vi "LIA Example FPGA.vi"() -> ()   [LabVIEW 2017]
uses:
  <instrlib>/_niInstr/Streaming/v1/Common/Stream State.ctl
  <instrlib>/_niInstr/Data Trigger/v1/Shared/Public/Edge Configuration FXP(+-,18,1).ctl
  <instrlib>/_niInstr/Data Trigger/v1/Shared/Public/Edge Configuration Trigger Slope.ctl
  <vilib>/Platform/TimedLoop/XDataNode/timing_clust.ctl
  <vilib>/Platform/TimedLoop/XDataNode/nitl_modes.ctl
  <vilib>/Platform/TimedLoop/XDataNode/wakeup.ctl
  <instrlib>/_niInstr/DSP/v1/Shared/Public/IQ Data.ctl
  <vilib>/rvi/Emulation/niFpgaSctlEmulationGetInTimedLoop.vi
  <vilib>/rvi/Emulation/niFpgaEmulationReportErrorSimple.vi
  <vilib>/rvi/Emulation/niFpgaGetClockAttributes.vi
  <vilib>/rvi/Emulation/niFpgaCriticalErrorInLSC.vi
  <instrlib>/_niInstr/DSP/v1/FPGA/Public/Sub VIs/Frequency Shift/Frequency Shift - 1 spc.vi
  <instrlib>/_niInstr/DSP/v1/FPGA/Public/Sub VIs/Fractional Decimator/Fractional Decimator - 1 spc - 2x oc.vi
  <userlib>/_NI Noise Generation IP/FPGA/Public/Low Level/AWGN FXP23x2.vi
  <instrlib>/_niInstr/DSP/v1/FPGA/Public/Sub VIs/Frequency Shift/Frequency Shift - 2 spc.vi
  <vilib>/rvi/eio/common/nirviEmuTemplateMethod_errors.vi
  <vilib>/Platform/TimedLoop/XDataNode/XDataNode.xnode
  <instrlib>/_niInstr/DSP/v1/Xnodes/Public/Frequency Shift/niInstr DSP v1 Frequency Shift FPGA.xnode
  <vilib>/rvi/FXPMathLib/FxpMul/XNode/nifxpmath_Multiplier.xnode
  <vilib>/rvi/FXPMathLib/FxpAdd/XNode/nifxpmath_Add.xnode
  <vilib>/eio/EIONode/EIONode.xnode
  <vilib>/Platform/TimedLoop/XDataNode/XDNodeRunTimeDep.lvlib
  <instrlib>/_niInstr/Basic Elements/v1/FPGA/niInstr Basic Elements v1 FPGA.lvlib
  <instrlib>/_niInstr/DSP/v1/Shared/niInstr DSP v1 Shared.lvlib
  <instrlib>/_niInstr/DSP/v1/FPGA/niInstr DSP v1 FPGA.lvlib
  Program Files (x86)/National Instruments/LabVIEW 2017/examples/Lock-In Amplifier/_NI PLL IP/FPGA/NI PLL IP FPGA.lvlib
  lib/fpga/Lock-In Amplifier Example FPGA.lvlib
  <instrlib>/_niInstr/Streaming/v1/Common/niInstr Streaming v1 Common.lvlib
  <userlib>/_NI Noise Generation IP/FPGA/NI Noise Generation IP FPGA v2.lvlib
  <vilib>/rvi/FXPMathLib/sim/FxpSim.dll
  <instrlib>/_niInstr/Data Trigger/v1/Shared/niInstr Data Trigger v1 Shared.lvlib
panel:
  in  "lock-in.fir fs":fxp<+,48,1>
  in  "lock-in.decimator 0":enum16{"CIC", "FIR"}(ring)
  in  "dpll.reset 1":bool
  in  "dpll.enable 1":bool
  in  "dpll.q 1":fxp<+,48,0>
  in  "dpll.m 1":i8
  in  "dpll.config 1":T1
  out "dpll.vco output 1":fxp<+/-,48,0>
  in  "dpll.channel 1":i32
  in  "dpll.channel 0":i32
  out "dpll.vco output 0":fxp<+/-,48,0>
  in  "dpll.config 0":T1
  in  "dpll.m 0":i8
  in  "dpll.q 0":fxp<+,48,0>
  in  "dpll.enable 0":bool
  in  "dpll.reset 0":bool
  in  "lock-in.enable 3":bool
  in  "lock-in.enable 2":bool
  in  "lock-in.enable 1":bool
  in  "lock-in.carrier 3":fxp<+/-,48,0>
  in  "lock-in.carrier 2":fxp<+/-,48,0>
  in  "lock-in.enable 0":bool
  in  "lock-in.channel select 3":i32
  in  "lock-in.carrier select 3":i32
  in  "lock-in.cic config valid 3":bool
  in  "lock-in.cic config 3":cluster{"factor":fxp<+,16,16>, "shift":i16}
  in  "lock-in.reset 3":bool
  out "stream.state 3":T3 caption="stream.state 0"
  out "stream.samples transferred 3":u64 caption="stream.samples transferred 0"
  out "stream.metadata 3":u64 caption="stream.metadata 0"
  in  "stream.num samples 3":u64 caption="stream.num samples 0"
  in  "stream.request state 3":T3 caption="stream.request state 0"
  in  "lock-in.channel select 2":i32
  in  "lock-in.carrier select 2":i32
  in  "lock-in.cic config valid 2":bool
  in  "lock-in.cic config 2":cluster{"factor":fxp<+,16,16>, "shift":i16}
  in  "lock-in.reset 2":bool
  out "stream.state 2":T3 caption="stream.state 0"
  out "stream.samples transferred 2":u64 caption="stream.samples transferred 0"
  out "stream.metadata 2":u64 caption="stream.metadata 0"
  in  "stream.num samples 2":u64 caption="stream.num samples 0"
  in  "stream.request state 2":T3 caption="stream.request state 0"
  out "pll.vco output 0":fxp<+/-,48,0>
  out "pll.vco output 1":fxp<+/-,48,0>
  out "stream.metadata 4":u64 caption="stream.metadata 0"
  out "stream.samples transferred 4":u64 caption="stream.samples transferred 0"
  out "stream.state 4":T3 caption="stream.state 0"
  in  "stream.request state 4":T3 caption="stream.request state 0"
  in  "stream.num samples 4":u64 caption="stream.num samples 0"
  in  "preview.channel select":i32
  in  "ao.reset 3":bool
  in  "ao.carrier 2":fxp<+/-,48,0>=0.010000000000001563
  in  "ao.level 2":fxp<+/-,18,1>
  in  "ao.reset 2":bool
  in  "ao.carrier 1":fxp<+/-,48,0>=0.010000000000001563
  in  "ao.level 1":fxp<+/-,18,1>
  in  "ao.reset 1":bool
  in  "ao.reset 0":bool
  in  "ao.carrier 0":fxp<+/-,48,0>=0.010000000000001563
  in  "ao.level 0":fxp<+/-,18,1>
  in  "lock-in.channel select 1":i32
  in  "lock-in.channel select 0":i32
  in  "stream.request state 1":T3 caption="stream.request state 0"
  in  "stream.num samples 1":u64 caption="stream.num samples 0"
  out "stream.metadata 1":u64 caption="stream.metadata 0"
  out "stream.samples transferred 1":u64 caption="stream.samples transferred 0"
  out "stream.state 1":T3 caption="stream.state 0"
  in  "lock-in.reset 1":bool
  in  "lock-in.cic config 1":cluster{"factor":fxp<+,16,16>, "shift":i16}
  in  "lock-in.cic config valid 1":bool
  in  "lock-in.carrier select 1":i32
  in  "lock-in.carrier select 0":i32
  in  "lock-in.cic config valid 0":bool
  in  "lock-in.cic config 0":cluster{"factor":fxp<+,16,16>, "shift":i16}
  in  "lock-in.reset 0":bool
  in  "lock-in.carrier 1":fxp<+/-,48,0>
  in  "lock-in.carrier 0":fxp<+/-,48,0>
  in  "ao.level 3":fxp<+/-,18,1>
  in  "pll.channel 1":i32
  in  "pll.reset 1":bool
  in  "pll.enable 1":bool
  in  "pll.config 1":T4={"quiescent frequency"=0.10000000000000142, "compensation"=0.0, "psd gain"=-18, "loop filter"={"order"=4, "cutoff"=6}}
  in  "pll.channel 0":i32
  in  "ao.noise gain 3":fxp<+,18,1>=0.01000213623046875
  in  "ao.carrier 3":fxp<+/-,48,0>=0.010000000000001563
  in  "ao.noise seeds 3":fxp<+,23,23>[](array[numeric])=[1.0, 12323.0]
  in  "pll.reset 0":bool
  in  "pll.enable 0":bool
  in  "stream.request state 0":T3
  in  "stream.num samples 0":u64
  out "stream.metadata 0":u64
  out "stream.samples transferred 0":u64
  out "stream.state 0":T3
  in  "pll.config 0":T4={"quiescent frequency"=0.10000000000000142, "compensation"=0.0, "psd gain"=-18, "loop filter"={"order"=4, "cutoff"=6}}
  out "IO Module\\InitDone":bool
  out "IO Module\\User Error":u32
  in  "IO Module\\User Command":u32
  in  "IO Module\\User Command Valid":bool
  out "IO Module\\User Command Ready":bool
  in  "IO Module\\User Command Arg 0":u32
  in  "IO Module\\User Command Arg 1":u32
  out "IO Module\\User Command Error":u16
  out "IO Module\\User Command Return":u32
  out "IO Module\\User Command Return Valid":bool
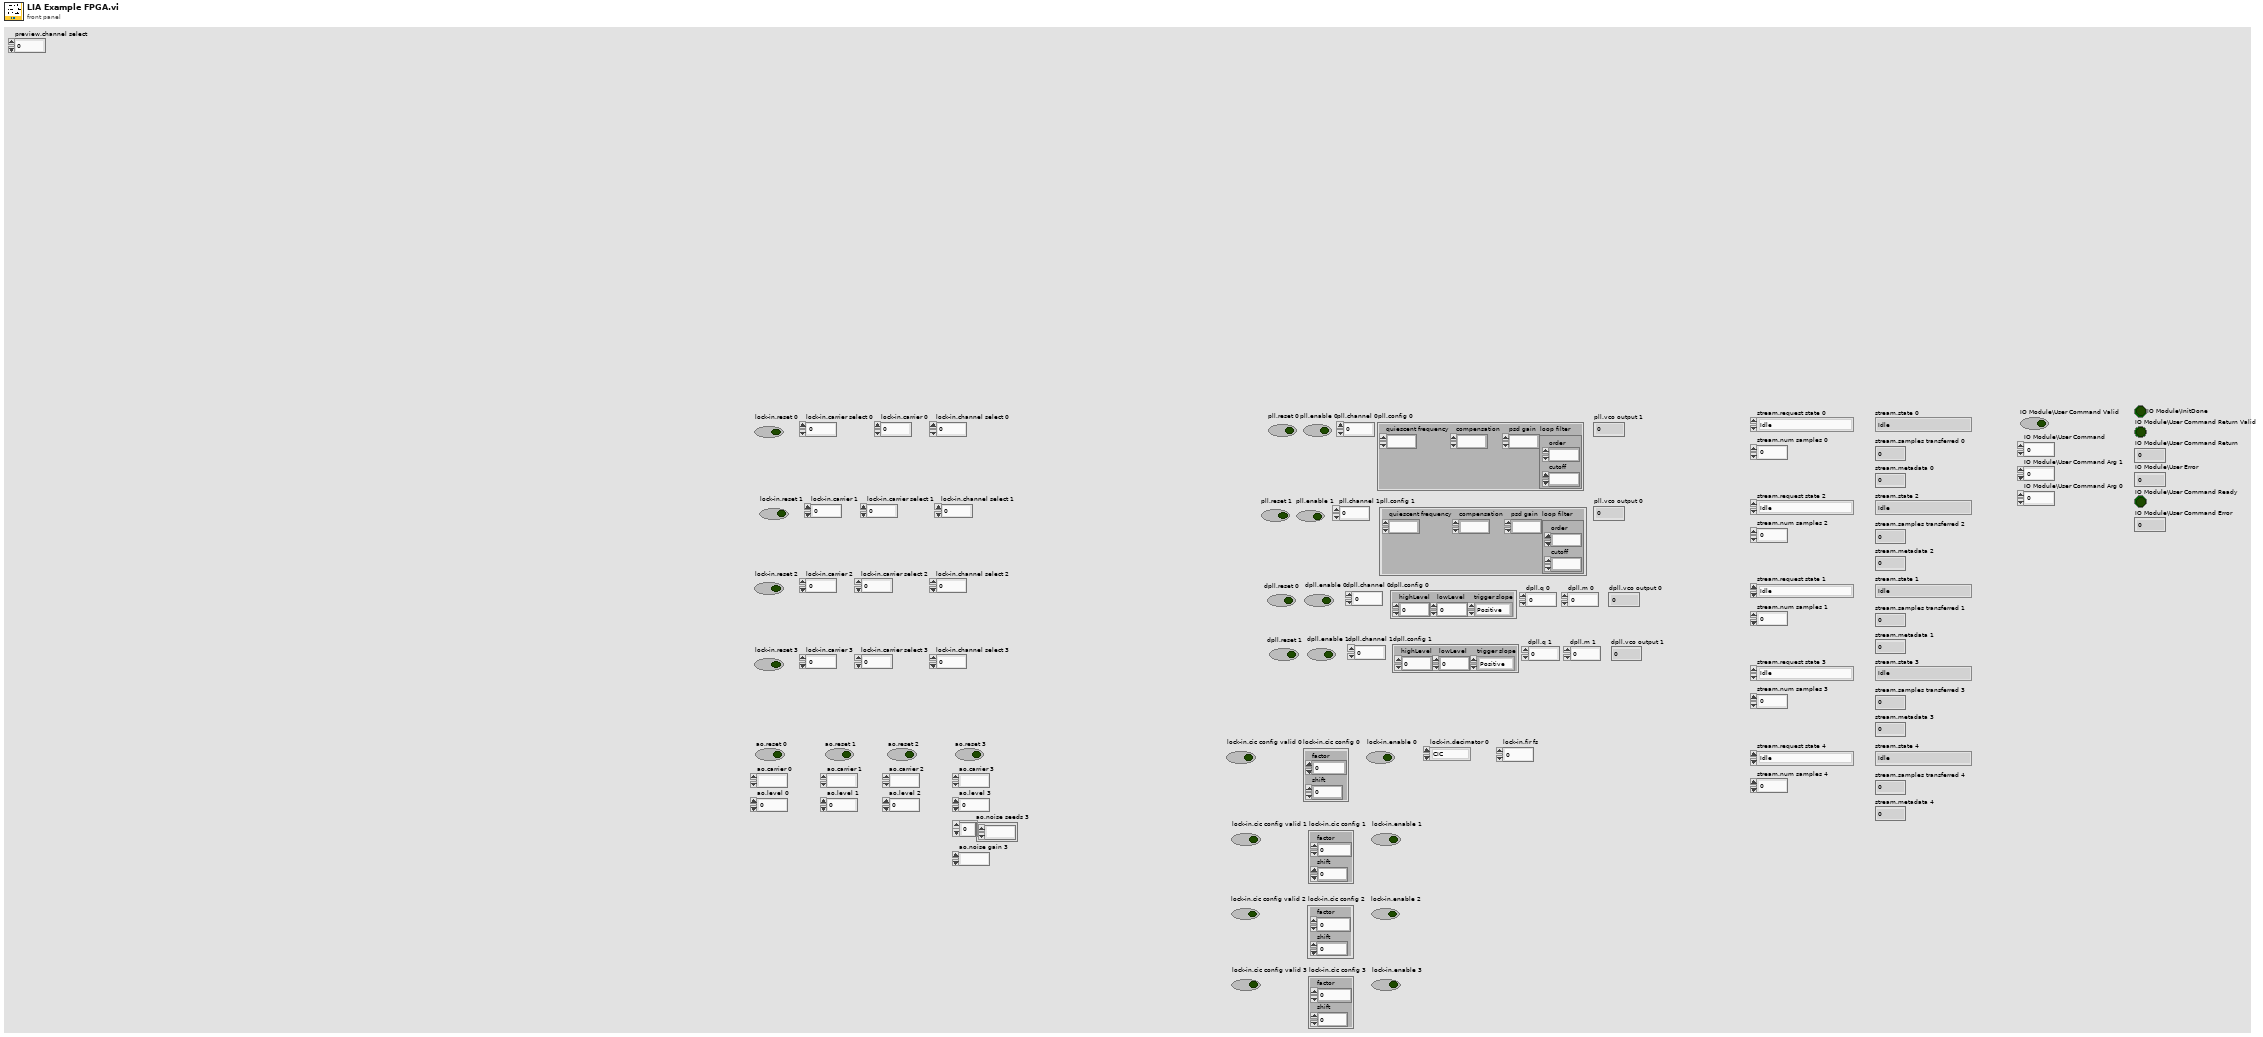
[diagram p1: front panel]
types:
  T1 = typedef "niInstr Data Trigger v1 Shared.lvlib/Edge Configuration FXP(+-,18,1).ctl" = cluster{"highLevel":fxp<+/-,18,1>, "lowLevel":fxp<+/-,18,1>, "trigger slope":T2}
  T2 = typedef "niInstr Data Trigger v1 Shared.lvlib/Edge Configuration Trigger Slope.ctl" = enum8{"Positive", "Negative"}
  T3 = typedef "niInstr Streaming v1 Common.lvlib/Stream State.ctl" = enum8{"Idle", "Finite Transfer", "Continuous", "Done", "Error", "Not Ready", "Cancel"}
  T4 = cluster{"quiescent frequency":fxp<+/-,48,0>, "compensation":fxp<+/-,18,3>, "psd gain":i16, "loop filter":cluster{"order":i32, "cutoff":i8}}
  T5 = typedef "XDNodeRunTimeDep.lvlib/timing_clust.ctl" = cluster{"Expected End [f-1]":u64, "Actual End [f-1]":u64, "Finished Late? [f-1]":bool, "Expected End [i-1]":u64, "Actual End [i-1]":u64, "Finished Late? [i-1]":bool, "Expected Start [i]":u64, "Actual Start [i]":u64, "Expected Start [f]":u64, "Actual Start [f]":u64, "Source Name":string, "Structure Name":string, "Period":i64, "Deadline":i64, "Offset":i64, "Start":i64, "Priority":i32, "Timeout":i32, "Mode":T6, "Wakeup Reason":T7, "Error":errorcluster, "Source Type":string, "Secondary Source Type":string, "Global End Time":u64, "Global Start Time":u64, "Frame Duration":u64, "Iteration Duration":u64, "Assigned CPU":i32, "I/O Scan Engine Mode":u32}
  T6 = typedef "XDNodeRunTimeDep.lvlib/nitl_modes.ctl" = enum32{"No Change", "Process missed periods, maintain original phase", "Discard missed periods, maintain original phase", "Process missed periods, ignore original phase", "Discard missed periods, ignore original phase"}
  T7 = typedef "XDNodeRunTimeDep.lvlib/wakeup.ctl" = enum32{"Normal", "Aborted", "Asynchronous wakeup", "Timing source error", "Timed loop error", "Timeout"}
  T8 = cluster{"stream.num samples 0":u64, "stream.request state 0":T3, "stream.index 0":i16}
  T9 = typedef "niInstr DSP v1 Shared.lvlib/IQ Data.ctl" = cluster{"I":fxp<+/-,18,1>, "Q":fxp<+/-,18,1>, "overflow":bool}
  T10 = cluster{"stream.metadata 0":u64, "stream.samples transferred 0":u64, "stream.state 0":T3}
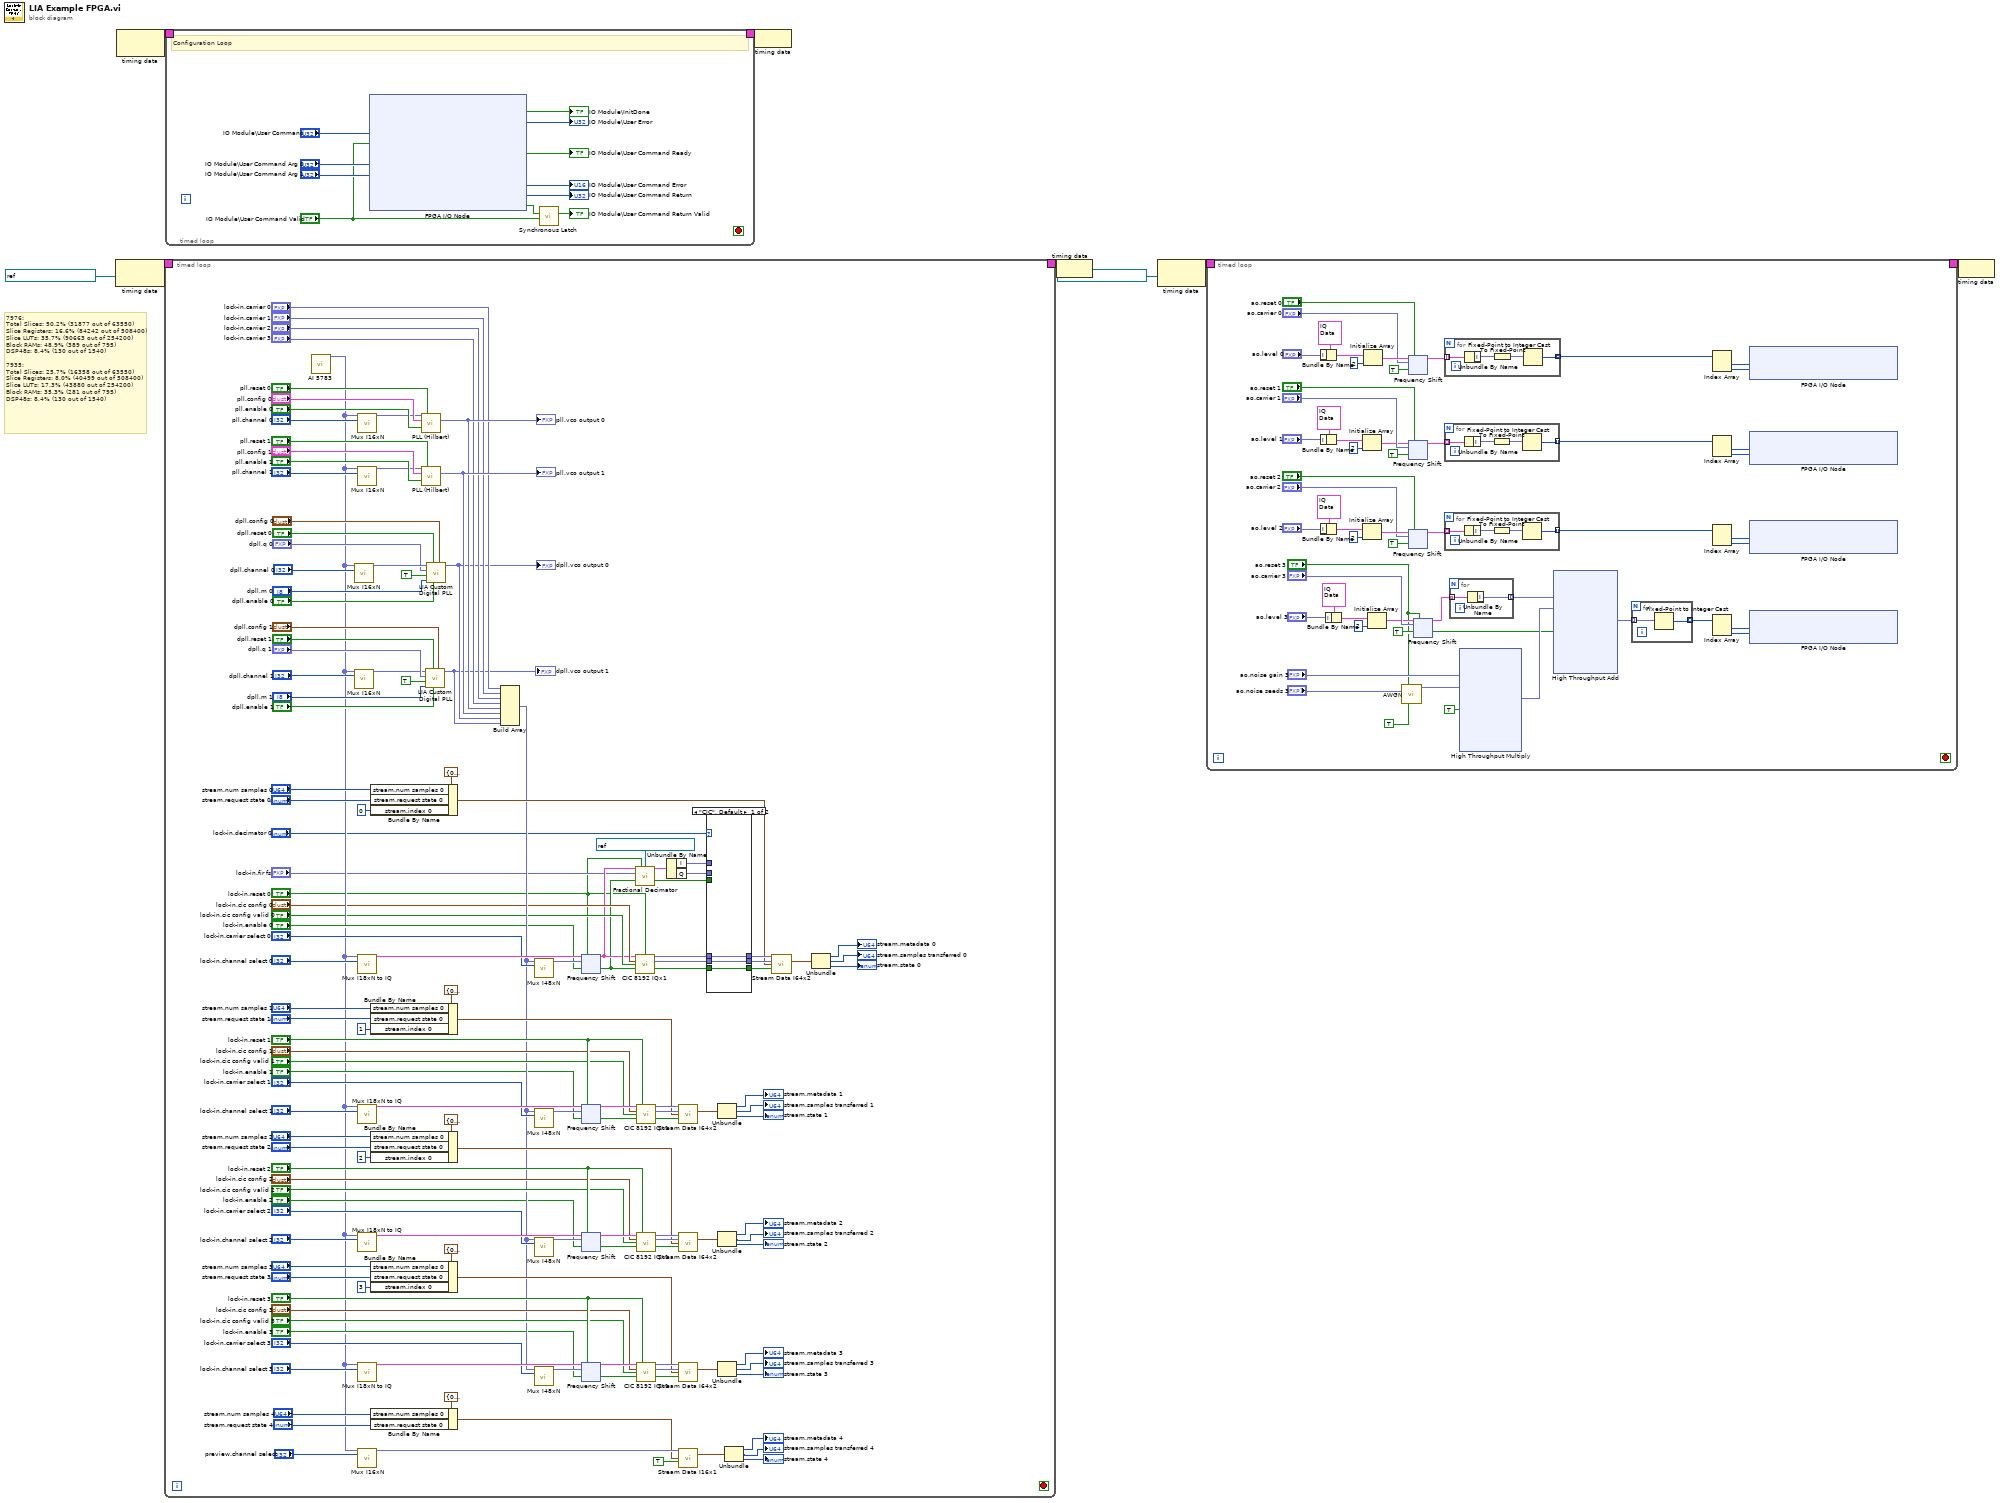
[diagram p0: block diagram]
diagram:
  # "7976:\nTotal Slices: 50.2% (31877 out of 63550)\nSlice Registers: 16.6% (84242 out of 508400)\nSlice LUTs: 35.7% (90663 out of 254200)\nBlock RAMs: 48.9% (389 out of 795)\nDSP48s: 8.4% (130 out of 1540)\n\n7935:\nTotal Slices: 25.7% (16358 out of 63550)\nSlice Registers: 8.0% (40499 out of 508400)\nSlice LUTs: 17.3% (43880 out of 254200)\nBlock RAMs: 35.3% (281 out of 795)\nDSP48s: 8.4% (130 out of 1540)"
  n1 = node-c288(refnum<k21> "IO Module\\Data Clock" ("Source Name")) -> (w8:T5)
  n2 = node-c288() -> (w2:T5)  [unwired: 1 in]
  n3 = timed-loop {
    timing: w8 -> [_]
    timing-out: [_] -> w7
    stop <- _ stop-if-true
    n4 = call "AI 5783.vi"() -> ("i18x1"=w25:fxp<+/-,18,1>[])  [unwired: 14 in, 1 out]
    n5 = call "Mux I16xN.vi"("i16xn in"=w25, "index"="dpll.channel 1") -> ("i16 out"=w28:fxp<+/-,18,1>)  [unwired: 12 in, 1 out]
    n6 = call "Mux I16xN.vi"("i16xn in"=w25, "index"="dpll.channel 0") -> ("i16 out"=w40:fxp<+/-,18,1>)  [unwired: 12 in, 1 out]
    n7 = call "Mux I16xN.vi"("i16xn in"=w25, "index"="pll.channel 0") -> ("i16 out"=w150:fxp<+/-,18,1>)  [unwired: 12 in, 1 out]
    n8 = call "Mux I16xN.vi"("i16xn in"=w25, "index"="pll.channel 1") -> ("i16 out"=w144:fxp<+/-,18,1>)  [unwired: 12 in, 1 out]
    n9 = call "Mux I18xN to IQ.vi"("i16xn in"=w25, "index"="lock-in.channel select 0") -> ("output"=w143:T9)  [unwired: 12 in, 1 out]
    n10 = call "Mux I18xN to IQ.vi"("i16xn in"=w25, "index"="lock-in.channel select 1") -> ("output"=w127:T9)  [unwired: 12 in, 1 out]
    n11 = call "Mux I18xN to IQ.vi"("i16xn in"=w25, "index"="lock-in.channel select 2") -> ("output"=w93:T9)  [unwired: 12 in, 1 out]
    n12 = call "Mux I18xN to IQ.vi"("i16xn in"=w25, "index"="lock-in.channel select 3") -> ("output"=w72:T9)  [unwired: 12 in, 1 out]
    n13 = call "Mux I16xN.vi"("i16xn in"=w25, "index"="preview.channel select") -> ("i16 out"=w101:fxp<+/-,18,1>)  [unwired: 12 in, 1 out]
    n14 = Bundle By Name(cluster=T8 {"stream.num samples 0"=0, "stream.request state 0"=enum."Idle", "stream.index 0"=0} ("config"), "stream.num samples 0"="stream.num samples 0", "stream.request state 0"="stream.request state 0", "stream.index 0"=i16 0) -> (w130:T8)
    n15 = Bundle By Name(cluster=T8 {"stream.num samples 0"=0, "stream.request state 0"=enum."Idle", "stream.index 0"=0} ("config"), "stream.num samples 0"="stream.num samples 1", "stream.request state 0"="stream.request state 1", "stream.index 0"=i16 1) -> (w109:T8)
    n16 = Bundle By Name(cluster=T8 {"stream.num samples 0"=0, "stream.request state 0"=enum."Idle", "stream.index 0"=0} ("config"), "stream.num samples 0"="stream.num samples 2", "stream.request state 0"="stream.request state 2", "stream.index 0"=i16 2) -> (w75:T8)
    n17 = Bundle By Name(cluster=T8 {"stream.num samples 0"=0, "stream.request state 0"=enum."Idle", "stream.index 0"=0} ("config"), "stream.num samples 0"="stream.num samples 3", "stream.request state 0"="stream.request state 3", "stream.index 0"=i16 3) -> (w54:T8)
    n18 = Bundle By Name(cluster=T8 {"stream.num samples 0"=0, "stream.request state 0"=enum."Idle", "stream.index 0"=0} ("config"), "stream.num samples 0"="stream.num samples 4", "stream.request state 0"="stream.request state 4") -> (w97:T8)
    n19 = call "PLL (Hilbert).vi"("input"=w150, "reset"="pll.reset 0", "config"="pll.config 0", "enable"="pll.enable 0") -> ("output"=w94:fxp<+/-,48,0>)  [unwired: 11 in]
    "pll.vco output 0" <- w94
    n20 = call "PLL (Hilbert).vi"("input"=w144, "reset"="pll.reset 1", "config"="pll.config 1", "enable"="pll.enable 1") -> ("output"=w95:fxp<+/-,48,0>)  [unwired: 11 in]
    "pll.vco output 1" <- w95
    n21 = call "LIA Custom Digital PLL.vi"("configuration"="dpll.config 1", "arm"="dpll.enable 1", "reset"="dpll.reset 1", "m"="dpll.m 1", "input valid"=TRUE, "q"="dpll.q 1", "I"=w28) -> ("frequency shift"=w24:fxp<+/-,48,0>)  [unwired: 1 in, 3 out]
    "dpll.vco output 1" <- w24
    n22 = call "LIA Custom Digital PLL.vi"("configuration"="dpll.config 0", "arm"="dpll.enable 0", "reset"="dpll.reset 0", "m"="dpll.m 0", "input valid"=TRUE, "q"="dpll.q 0", "I"=w40) -> ("frequency shift"=w35:fxp<+/-,48,0>)  [unwired: 1 in, 3 out]
    "dpll.vco output 0" <- w35
    n23 = Build Array("lock-in.carrier 0", "lock-in.carrier 1", "lock-in.carrier 2", "lock-in.carrier 3", w94, w95, w35, w24) -> (w51:fxp<+/-,48,0>[])
    n24 = call "Mux I48xN.vi"("i48xn in"=w51, "index"="lock-in.carrier select 0") -> ("i48 out"=w142:fxp<+/-,48,0>)  [unwired: 13 in]
    n25 = call "Mux I48xN.vi"("i48xn in"=w51, "index"="lock-in.carrier select 1") -> ("i48 out"=w126:fxp<+/-,48,0>)  [unwired: 13 in]
    n26 = call "Mux I48xN.vi"("i48xn in"=w51, "index"="lock-in.carrier select 2") -> ("i48 out"=w92:fxp<+/-,48,0>)  [unwired: 13 in]
    n27 = call "Mux I48xN.vi"("i48xn in"=w51, "index"="lock-in.carrier select 3") -> ("i48 out"=w71:fxp<+/-,48,0>)  [unwired: 13 in]
    n28 = xnode "Frequency Shift"("data in"=w143, "reset"="lock-in.reset 0", "frequency shift"=w142, "input valid"="lock-in.enable 0") -> ("data out"=w18:T9, "output valid"=w13:bool)  [unwired: 2 in, 1 out]
    n29 = xnode "Frequency Shift"("data in"=w127, "reset"="lock-in.reset 1", "frequency shift"=w126, "input valid"="lock-in.enable 1") -> ("data out"=w125:T9, "output valid"=w124:bool)  [unwired: 2 in, 1 out]
    n30 = xnode "Frequency Shift"("data in"=w93, "reset"="lock-in.reset 2", "frequency shift"=w92, "input valid"="lock-in.enable 2") -> ("data out"=w91:T9, "output valid"=w90:bool)  [unwired: 2 in, 1 out]
    n31 = xnode "Frequency Shift"("data in"=w72, "reset"="lock-in.reset 3", "frequency shift"=w71, "input valid"="lock-in.enable 3") -> ("data out"=w70:T9, "output valid"=w69:bool)  [unwired: 2 in, 1 out]
    n32 = call-poly <instrlib>:"Fractional Decimator.vi"("data in"=w18, "reset"="lock-in.reset 0", "clock x 2"=refnum<k21> "IO Module\\Data Clock 2x", "output sample rate"="lock-in.fir fs", "input valid"=w13) -> ("data out"=w21:T9, "output valid"=w10:bool)  [unwired: 8 in, 1 out]
    n33 = call "CIC 8192 IQx1.vi"("data"=w18, "reset"="lock-in.reset 0", "config"="lock-in.cic config 0", "config valid"="lock-in.cic config valid 0", "input valid"=w13) -> ("i out"=w17:fxp<+/-,64,1>, "q out"=w16:fxp<+/-,64,1>, "output valid"=w15:bool)  [unwired: 8 in]
    n34 = call "CIC 8192 IQx1.vi"("data"=w125, "reset"="lock-in.reset 1", "config"="lock-in.cic config 1", "config valid"="lock-in.cic config valid 1", "input valid"=w124) -> ("i out"=w120:fxp<+/-,64,1>, "q out"=w119:fxp<+/-,64,1>, "output valid"=w118:bool)  [unwired: 8 in]
    n35 = call "CIC 8192 IQx1.vi"("data"=w91, "reset"="lock-in.reset 2", "config"="lock-in.cic config 2", "config valid"="lock-in.cic config valid 2", "input valid"=w90) -> ("i out"=w86:fxp<+/-,64,1>, "q out"=w85:fxp<+/-,64,1>, "output valid"=w84:bool)  [unwired: 8 in]
    n36 = call "CIC 8192 IQx1.vi"("data"=w70, "reset"="lock-in.reset 3", "config"="lock-in.cic config 3", "config valid"="lock-in.cic config valid 3", "input valid"=w69) -> ("i out"=w65:fxp<+/-,64,1>, "q out"=w64:fxp<+/-,64,1>, "output valid"=w63:bool)  [unwired: 8 in]
    n37 = Unbundle By Name(w21) -> ("I"=w11:fxp<+/-,18,1>, "Q"=w9:fxp<+/-,18,1>)
    n38 = call "Stream Data I64x2.vi"("i in"=w120, "q in"=w119, "config"=w109, "input valid"=w118) -> ("status"=w117:T10)  [unwired: 11 in]
    n39 = call "Stream Data I64x2.vi"("i in"=w86, "q in"=w85, "config"=w75, "input valid"=w84) -> ("status"=w83:T10)  [unwired: 11 in]
    n40 = call "Stream Data I64x2.vi"("i in"=w65, "q in"=w64, "config"=w54, "input valid"=w63) -> ("status"=w62:T10)  [unwired: 11 in]
    n41 = call "Stream Data I16x1.vi"("i in"=w101, "config"=w97, "input valid"=TRUE) -> ("status"=w103:T10)  [unwired: 12 in]
    n42 = case shown="\"CIC\", Default" "lock-in.decimator 0" {
      tunnel: [w156 w159] -> w141
      tunnel: [w155 w158] -> w140
      tunnel: [w154 w157] -> w139
      tunnel: w17 -> [w156 _]
      tunnel: w16 -> [w155 _]
      tunnel: w15 -> [w154 _]
      tunnel: w11 -> [_ w159]
      tunnel: w10 -> [_ w157]
      tunnel: w9 -> [_ w158]
      frame "CIC", Default {
      }
      frame "FIR" {
      }
    }
    n43 = Unbundle(w117) -> ("stream.metadata 0"=→"stream.metadata 1":u64, "stream.samples transferred 0"=→"stream.samples transferred 1":u64, "stream.state 0"=→"stream.state 1":T3)
    n44 = Unbundle(w83) -> ("stream.metadata 0"=→"stream.metadata 2":u64, "stream.samples transferred 0"=→"stream.samples transferred 2":u64, "stream.state 0"=→"stream.state 2":T3)
    n45 = Unbundle(w62) -> ("stream.metadata 0"=→"stream.metadata 3":u64, "stream.samples transferred 0"=→"stream.samples transferred 3":u64, "stream.state 0"=→"stream.state 3":T3)
    n46 = Unbundle(w103) -> ("stream.metadata 0"=→"stream.metadata 4":u64, "stream.samples transferred 0"=→"stream.samples transferred 4":u64, "stream.state 0"=→"stream.state 4":T3)
    n47 = call "Stream Data I64x2.vi"("i in"=w141, "q in"=w140, "config"=w130, "input valid"=w139) -> ("status"=w138:T10)  [unwired: 11 in]
    n48 = Unbundle(w138) -> ("stream.metadata 0"=→"stream.metadata 0":u64, "stream.samples transferred 0"=→"stream.samples transferred 0":u64, "stream.state 0"=→"stream.state 0":T3)
  }
  n49 = timed-loop {
    timing: w2 -> [_]
    timing-out: [_] -> w1
    stop <- _ stop-if-true
    # "Configuration Loop"
    n50 = xnode "FPGA I/O Node"("IO Module\\User Command"="IO Module\\User Command", "IO Module\\User Command Valid"="IO Module\\User Command Valid", "IO Module\\User Command Arg 0"="IO Module\\User Command Arg 0", "IO Module\\User Command Arg 1"="IO Module\\User Command Arg 1") -> ("IO Module\\InitDone"=→"IO Module\\InitDone":bool, "IO Module\\Clip Error Code"=→"IO Module\\User Error":u32, "IO Module\\User Command Ready"=→"IO Module\\User Command Ready":bool, "IO Module\\User Command Error"=→"IO Module\\User Command Error":u16, "IO Module\\User Command Return"=→"IO Module\\User Command Return":u32, "IO Module\\User Command Return Valid"=w199:bool)  [unwired: 10 in, 10 out]
    n51 = call <instrlib>:"Synchronous Latch.vi"("clear"="IO Module\\User Command Valid", "set"=w199) -> ("out"=→"IO Module\\User Command Return Valid":bool)  [unwired: 9 in]
  }
  n52 = node-c288(w1) -> ()
  n53 = node-c288(w7) -> ()
  n54 = node-c288(refnum<k21> "IO Module\\Data Clock" ("Source Name")) -> (w5:T5)
  n55 = timed-loop {
    timing: w5 -> [_]
    timing-out: [_] -> w4
    stop <- _ stop-if-true
    n56 = Bundle By Name(cluster=T9 {"I"=0.0, "Q"=0.0, "overflow"=FALSE} ("output"), "I"="ao.level 1") -> (w232:T9)
    n57 = Bundle By Name(cluster=T9 {"I"=0.0, "Q"=0.0, "overflow"=FALSE} ("output"), "I"="ao.level 2") -> (w222:T9)
    n58 = Bundle By Name(cluster=T9 {"I"=0.0, "Q"=0.0, "overflow"=FALSE} ("output"), "I"="ao.level 0") -> (w247:T9)
    n59 = Bundle By Name(cluster=T9 {"I"=0.0, "Q"=0.0, "overflow"=FALSE} ("output"), "I"="ao.level 3") -> (w256:T9)
    n60 = Initialize Array(w232, 2 ("dimension size")) -> (w228:T9[])
    n61 = Initialize Array(w222, 2 ("dimension size")) -> (w226:T9[])
    n62 = Initialize Array(w247, 2 ("dimension size")) -> (w251:T9[])
    n63 = Initialize Array(w256, 2 ("dimension size")) -> (w252:T9[])
    n64 = call-poly <userlib>:"AWGN.vi"("reset"="ao.reset 3", "seeds"="ao.noise seeds 3", "ready"=TRUE) -> ("output 0"=w259:fxp<+/-,23,4>[])  [unwired: 10 in, 2 out]
    n65 = xnode "Frequency Shift"("data in"=w228, "reset"="ao.reset 1", "frequency shift"="ao.carrier 1", "input valid"=TRUE) -> ("data out"=w236:T9[])  [unwired: 2 in, 2 out]
    n66 = xnode "Frequency Shift"("data in"=w226, "reset"="ao.reset 2", "frequency shift"="ao.carrier 2", "input valid"=TRUE) -> ("data out"=w218:T9[])  [unwired: 2 in, 2 out]
    n67 = xnode "Frequency Shift"("data in"=w251, "reset"="ao.reset 0", "frequency shift"="ao.carrier 0", "input valid"=TRUE) -> ("data out"=w243:T9[])  [unwired: 2 in, 2 out]
    n68 = xnode "Frequency Shift"("data in"=w252, "reset"="ao.reset 3", "frequency shift"="ao.carrier 3", "input valid"=TRUE) -> ("data out"=w267:T9[], "output valid"=w264:bool)  [unwired: 2 in, 1 out]
    n69 = for {
      tunnel: w236 -> [w283] mode=indexing
      tunnel: [w284] -> w237 mode=indexing
      n70 = Unbundle By Name(w283) -> ("I"=w282:fxp<+/-,18,1>)
      n71 = To Fixed-Point(number=w282) -> (fixed-point=w281:fxp<+/-,16,1>)  [unwired: 1 in]
      n72 = Fixed-Point to Integer Cast(1:w281) -> (0:w284:i16)
    }
    n73 = for {
      tunnel: w218 -> [w270] mode=indexing
      tunnel: [w271] -> w217 mode=indexing
      n74 = Unbundle By Name(w270) -> ("I"=w269:fxp<+/-,18,1>)
      n75 = To Fixed-Point(number=w269) -> (fixed-point=w268:fxp<+/-,16,1>)  [unwired: 1 in]
      n76 = Fixed-Point to Integer Cast(1:w268) -> (0:w271:i16)
    }
    n77 = for {
      tunnel: w243 -> [w296] mode=indexing
      tunnel: [w297] -> w242 mode=indexing
      n78 = Unbundle By Name(w296) -> ("I"=w295:fxp<+/-,18,1>)
      n79 = To Fixed-Point(number=w295) -> (fixed-point=w294:fxp<+/-,16,1>)  [unwired: 1 in]
      n80 = Fixed-Point to Integer Cast(1:w294) -> (0:w297:i16)
    }
    n81 = for {
      tunnel: w267 -> [w310] mode=indexing
      tunnel: [w309] -> w263 mode=indexing
      n82 = Unbundle By Name(w310) -> ("I"=w309:fxp<+/-,18,1>)
    }
    n83 = xnode ("High Throughput Multiply")("x"="ao.noise gain 3", "y"=w259, "input valid"=TRUE) -> ("x*y"=w266:fxp<+/-,41,5>[])  [unwired: 1 in, 2 out]
    n84 = xnode ("High Throughput Add")("x"=w263, "y"=w266, "input valid"=w264) -> ("x+y"=w258:fxp<+/-,16,1>[])  [unwired: 1 in, 2 out]
    n85 = for {
      tunnel: w258 -> [w308] mode=indexing
      tunnel: [w307] -> w227 mode=indexing
      n86 = Fixed-Point to Integer Cast(1:w308) -> (0:w307:i16)
    }
    n87 = Index Array(array=w242) -> (element #1=w241:i16, element #2=w240:i16)  [unwired: 2 in]
    n88 = Index Array(array=w237) -> (element #1=w238:i16, element #2=w239:i16)  [unwired: 2 in]
    n89 = Index Array(array=w217) -> (element #1=w216:i16, element #2=w215:i16)  [unwired: 2 in]
    n90 = Index Array(array=w227) -> (element #1=w214:i16, element #2=w213:i16)  [unwired: 2 in]
    n91 = xnode "FPGA I/O Node"("IO Module\\AO 1 Data N-1 Data Clock"=w238, "IO Module\\AO 1 Data N Data Clock"=w239) -> ()  [unwired: 2 in, 2 out]
    n92 = xnode "FPGA I/O Node"("IO Module\\AO 2 Data N-1 Data Clock"=w216, "IO Module\\AO 2 Data N Data Clock"=w215) -> ()  [unwired: 2 in, 2 out]
    n93 = xnode "FPGA I/O Node"("IO Module\\AO 3 Data N-1 Data Clock"=w214, "IO Module\\AO 3 Data N Data Clock"=w213) -> ()  [unwired: 2 in, 2 out]
    n94 = xnode "FPGA I/O Node"("IO Module\\AO 0 Data N-1 Data Clock"=w241, "IO Module\\AO 0 Data N Data Clock"=w240) -> ()  [unwired: 2 in, 2 out]
  }
  n95 = node-c288(w4) -> ()
